vi "Read Configuration Class Name.vi"(8 "error in":errorcluster, 11 "CVT editor node in":refnum<class "CVT editor node.lvclass">) -> (0 "error out":errorcluster, 2 "Class Name":string, 3 "CVT editor node out":refnum<class "CVT editor node.lvclass">)   [LabVIEW 2013, in "CVT editor node.lvclass"]
uses:
  CVT editor node.lvclass
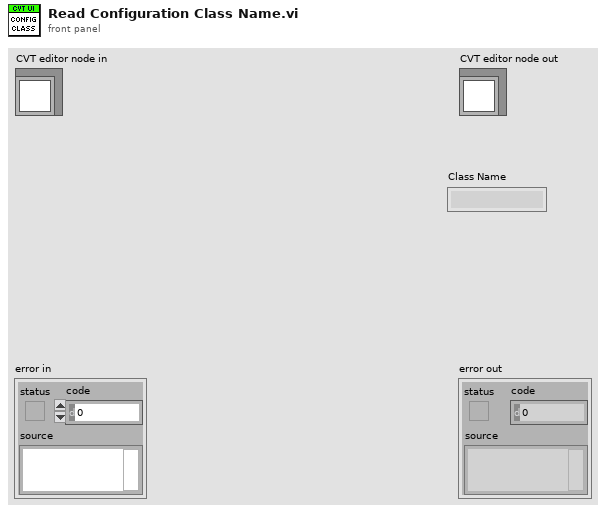
[diagram p1: front panel]
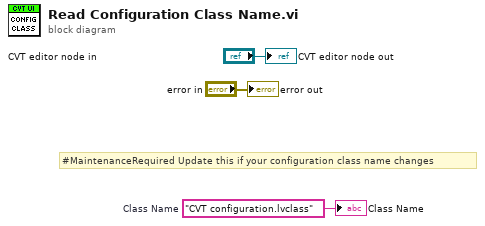
[diagram p0: block diagram]
diagram:
  w1 = "CVT configuration.lvclass"  # Class Name
  # "#MaintenanceRequired Update this if your configuration class name changes"
  "error out" <- "error in"
  "CVT editor node out" <- "CVT editor node in"
  "Class Name" <- w1
